vi "Create Network Stream Writer.vi"(8 "error in (no error)":errorcluster) -> (0 "error out":errorcluster, 3 "RT writer":refnum<k21>)   [LabVIEW 2024]
uses:
  <vilib>/dex/Stream Element Allocation Mode.ctl
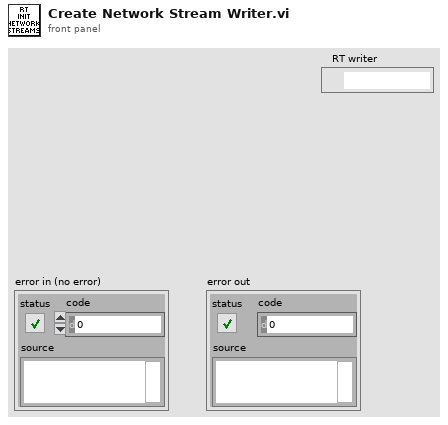
[diagram p1: front panel]
types:
  T1 = typedef "Stream Element Allocation Mode.ctl" = u32
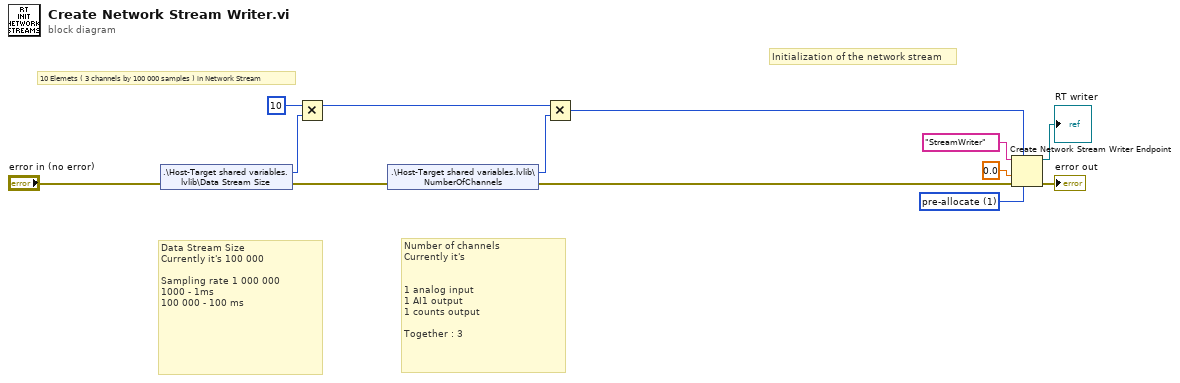
[diagram p0: block diagram]
diagram:
  w11 = T1 1 items=["allocate as needed", "pre-allocate"] ("element allocation mode")
  # "10 Elemets ( 3 channels by 100 000 samples ) in Network Stream"
  # "Data Stream Size\nCurrently it's 100 000\n\nSampling rate 1 000 000\n1000 - 1ms\n100 000 - 100 ms"
  # "Number of channels\nCurrently it's\n\n\n1 analog input \n1 AI1 output\n1 counts output\n\nTogether : 3"
  # "Initialization of the network stream"
  n1 = shared-variable ".\\Host-Target shared variables.lvlib\\Data Stream Size"(error in="error in (no error)") -> (w2:u32, error out=w4:errorcluster)
  n2 = Multiply(x=u32 10, y=w2) -> (x*y=w3:u32)
  n3 = shared-variable ".\\Host-Target shared variables.lvlib\\NumberOfChannels"(error in=w4) -> (w9:u8, error out=w7:errorcluster)
  n4 = Multiply(x=w3, y=w9) -> (x*y=w8:u32)
  n5 = Create Network Stream Writer Endpoint(6:w11, 7:w8, 8:w7, 9:sgl 0.0, 11:"StreamWriter" ("writer name")) -> (0:→"error out":errorcluster, 3:→"RT writer":refnum<k21>)  [unwired: 2 in]
